vi "LookCANFileInfo.vi"(0 "Path输入":refnum<vi>, 1 "Language":u32, 2 "CAN报文统计":refnum<vi>, 3 "DBC数组":refnum<vi>) -> ()   [LabVIEW 2015]
panel:
  out "txtTile":string="CAN离线数据文件详细信息"
  out "文件信息":string
  out "报文统计":string[][](array[string])
  # "CAN离线数据文件详细信息"
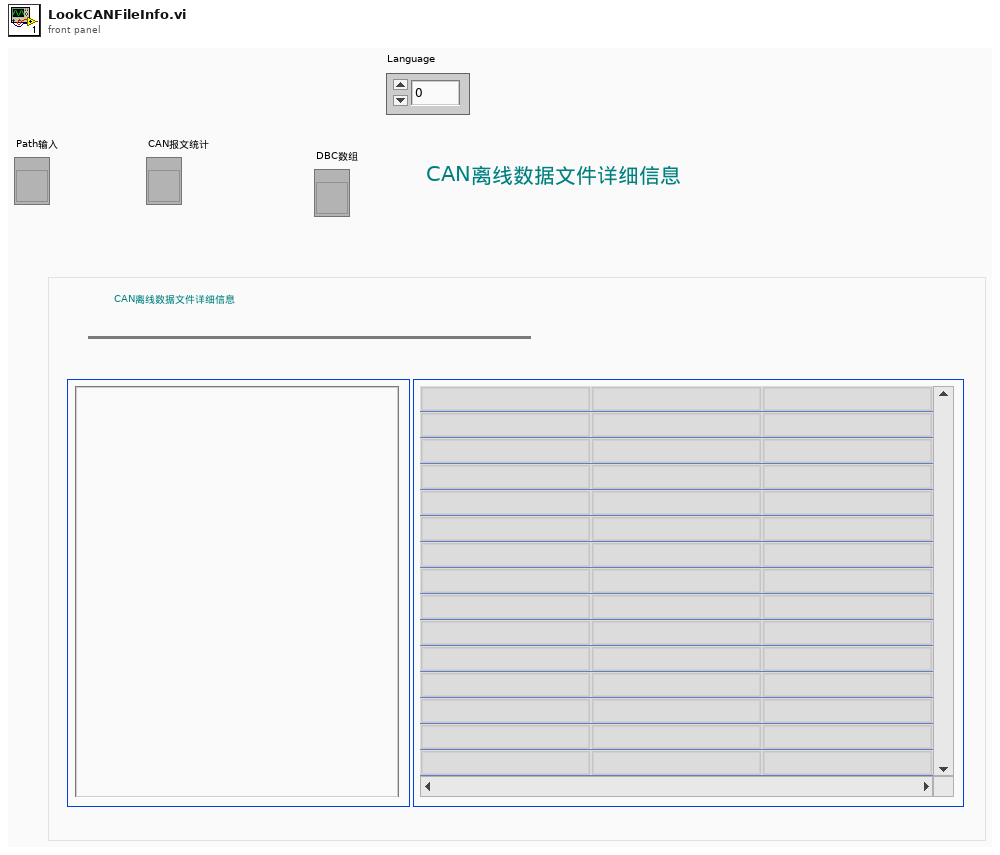
[diagram p1: front panel]
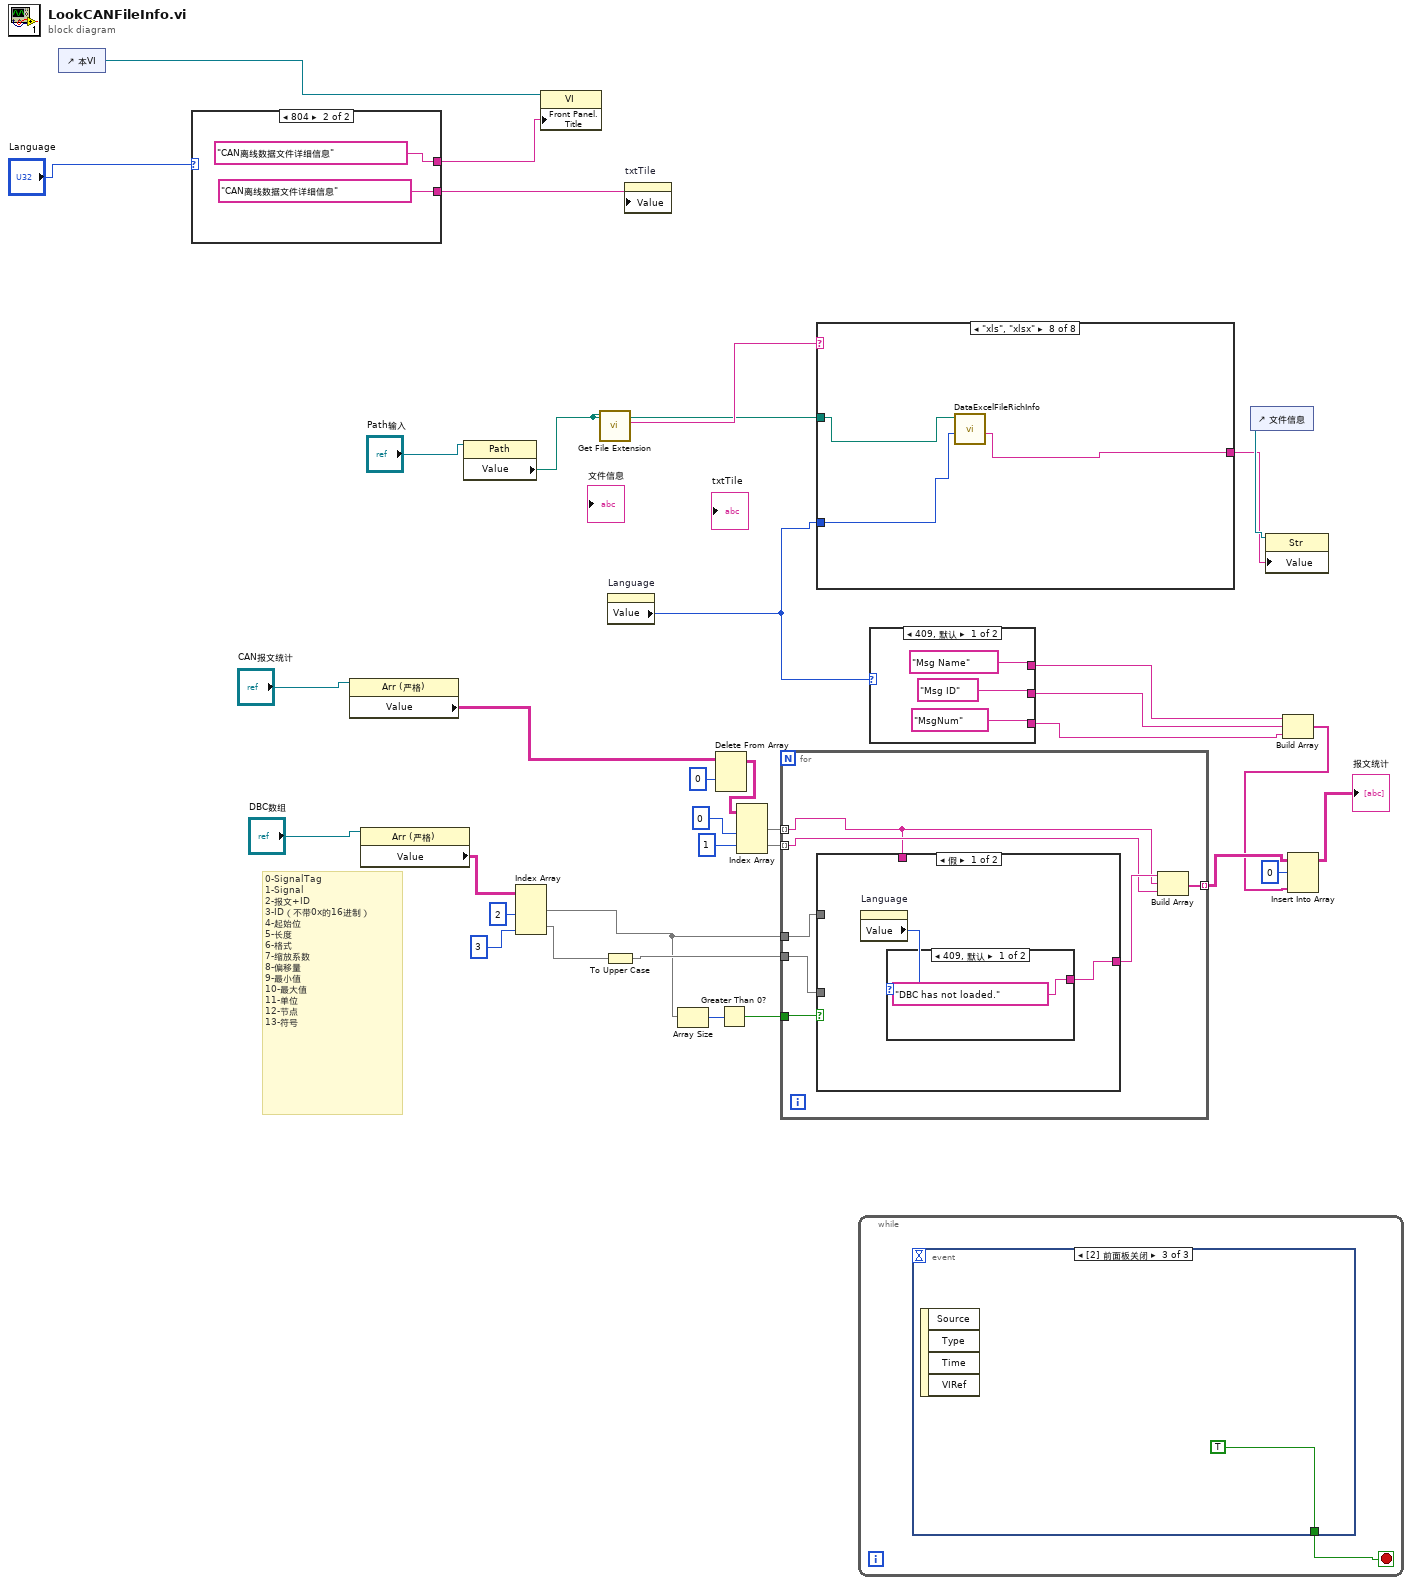
[diagram p0: block diagram]
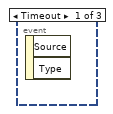
[diagram p2: hidden frame]
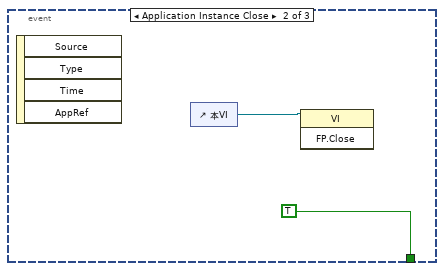
[diagram p3: hidden frame]
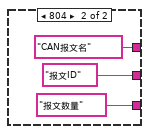
[diagram p4: hidden frame]
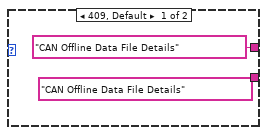
[diagram p5: hidden frame]
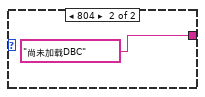
[diagram p6: hidden frame]
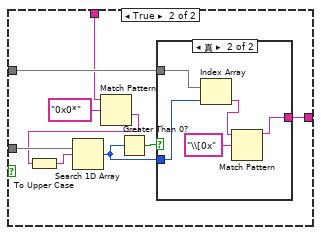
[diagram p7: hidden frame]
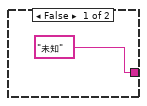
[diagram p8: hidden frame]
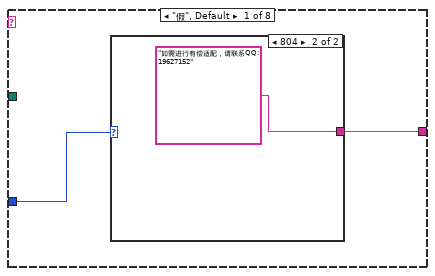
[diagram p9: hidden frame]
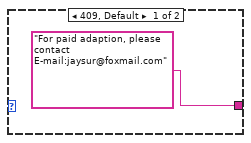
[diagram p10: hidden frame]
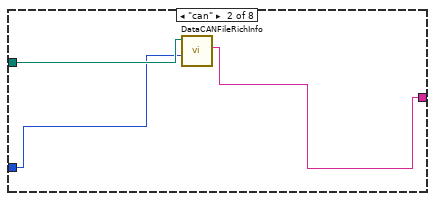
[diagram p11: hidden frame]
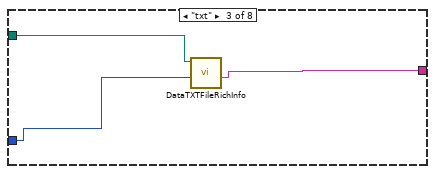
[diagram p12: hidden frame]
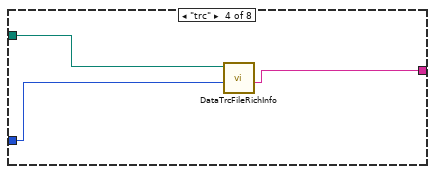
[diagram p13: hidden frame]
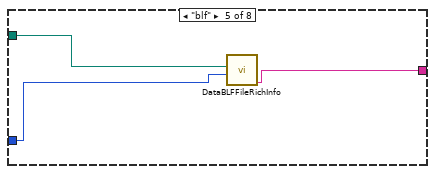
[diagram p14: hidden frame]
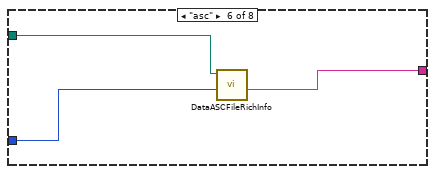
[diagram p15: hidden frame]
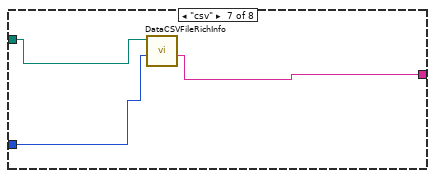
[diagram p16: hidden frame]
diagram:
  # "0-SignalTag\n1-Signal\n2-报文+ID\n3-ID（不带0x的16进制）\n4-起始位\n5-长度\n6-格式\n7-缩放系数\n8-偏移量\n9-最小值\n10-最大值\n11-单位\n12-节点\n13-符号"
  n1 = control-ref of="本VI"() -> (w2:refnum<vi>)
  n2 = case shown="804" "Language" {
    tunnel: ["CAN Offline Data File Details" "CAN离线数据文件详细信息"] -> w4
    tunnel: ["CAN Offline Data File Details" "CAN离线数据文件详细信息"] -> w1
    frame 409, Default {
    }
    frame 804 {
    }
  }
  n3 = property class="Arr (严格)"(reference="CAN报文统计") -> ("Value"=w23:string[][])  [unwired: 1 in, 2 out]
  n4 = property class="Arr (严格)"(reference="DBC数组") -> ("Value"=w27:string[][])  [unwired: 1 in, 2 out]
  n5 = property class="Path"(reference="Path输入") -> ("Value"=w31:path)  [unwired: 1 in, 2 out]
  n6 = Index Array(array=w27, index (col) #1=2 ("禁用的索引 (列)"), index (col) #2=3 ("索引 (列)")) -> (element #1=w20:string[], element #2=w22:string[])  [unwired: 2 in]
  n7 = property class="VI"(reference=w2, "Front Panel.Title"=w1) -> ()  [unwired: 1 in, 2 out]
  n8 = call <vilib>:"Get File Extension.vi"("file"=w31) -> ("lowercase file extension"=w32:string)  [unwired: 6 in, 4 out]
  n9 = To Upper Case(1:w22) -> (0:w21:string[])
  n10 = property on="Language" class="DigNum (严格)"() -> ("Value"=w3:u32)  [unwired: 2 in, 2 out]
  n11 = property on="txtTile" class="Str"("Value"=w4) -> ()  [unwired: 2 in, 2 out]
  n12 = Array Size(array=w20) -> (size(s)=w24:i32)
  n13 = Delete From Array(array=w23, index (row)=0 ("索引 (行)")) -> (array with subset deleted=w17:string[][])  [unwired: 2 in, 1 out]
  n14 = Greater Than 0?(x=w24) -> (x > 0?=w8:bool)
  n15 = Index Array(array=w17, index (col) #1=0 ("禁用的索引 (列)"), index (col) #2=1 ("索引 (列)")) -> (element #1=w14:string[], element #2=w13:string[])  [unwired: 2 in]
  n16 = for {
    tunnel: w14 -> [w39] mode=indexing
    tunnel: w13 -> [w41] mode=indexing
    tunnel: w20 -> [w45]
    tunnel: w21 -> [w44]
    tunnel: [w42] -> w12 mode=indexing
    tunnel: w8 -> [w40]
    n17 = case shown="假" w40 {
      tunnel: w45 -> [_ w58]
      tunnel: w44 -> [_ w57]
      tunnel: [w47 w56] -> w43
      tunnel: w39 -> [_ w54]
      frame False {
        n18 = property on="Language" class="DigNum (严格)"() -> ("Value"=w46:u32)  [unwired: 2 in, 2 out]
        n19 = case shown="409, 默认" w46 {
          tunnel: ["DBC has not loaded." "尚未加载DBC"] -> w47
          frame 409, Default {
          }
          frame 804 {
          }
        }
      }
      frame True {
        n20 = Match Pattern(string=w54, regular expression="0x0*" ("正则表达式")) -> (after substring=w50:string)  [unwired: 1 in, 3 out]
        n21 = To Upper Case(1:w50) -> (0:w51:string)
        n22 = Search 1D Array(1D array=w57, element=w51) -> (index of element=w52:i32)  [unwired: 1 in]
        n23 = Greater Than 0?(x=w52) -> (x > 0?=w55:bool)
        n24 = case shown="真" w55 {
          tunnel: w58 -> [_ w64]
          tunnel: ["未知" w61] -> w56
          tunnel: w52 -> [_ w63]
          frame False {
          }
          frame True {
            n25 = Index Array(array=w64, index=w63) -> (element=w62:string)
            n26 = Match Pattern(string=w62, regular expression="\\[0x" ("正则表达式")) -> (before substring=w61:string)  [unwired: 1 in, 3 out]
          }
        }
      }
    }
    n27 = Build Array(w43, w39, w41) -> (w42:string[])
  }
  n28 = case shown="\"xls\", \"xlsx\"" w32 {
    tunnel: w31 -> [_ w70 w74 w77 w79 w83 w86 w89]
    tunnel: [w66 w71 w73 w75 w78 w82 w85 w88] -> w29
    tunnel: w3 -> [w65 w69 w72 w76 w80 w81 w84 w87]
    frame "假", Default {
      n29 = case shown="804" w65 {
        tunnel: ["For paid adaption, please contact E-mail:jaysur@foxmail.com" "如需进行有偿适配，请联系QQ:19627152"] -> w66
        frame 409, Default {
        }
        frame 804 {
        }
      }
    }
    frame "can" {
      n30 = call "DataCANFileRichInfo.vi"("Language"=w69, "file path (dialog if empty)"=w70) -> ("FileInfo"=w71:string)  [unwired: 7 in, 2 out]
    }
    frame "txt" {
      n31 = call "DataTXTFileRichInfo.vi"("Language"=w72, "file path (dialog if empty)"=w74) -> ("FileInfo"=w73:string)  [unwired: 7 in, 2 out]
    }
    frame "trc" {
      n32 = call "DataTrcFileRichInfo.vi"("Language"=w76, "file path (dialog if empty)"=w77) -> ("FileInfo"=w75:string)  [unwired: 7 in, 2 out]
    }
    frame "blf" {
      n33 = call "DataBLFFileRichInfo.vi"("Language"=w80, "file path (dialog if empty)"=w79) -> ("FileInfo"=w78:string)  [unwired: 7 in, 2 out]
    }
    frame "asc" {
      n34 = call "DataASCFileRichInfo.vi"("Language"=w81, "file path (dialog if empty)"=w83) -> ("FileInfo"=w82:string)  [unwired: 7 in, 2 out]
    }
    frame "csv" {
      n35 = call "DataCSVFileRichInfo.vi"("Language"=w84, "file path (dialog if empty)"=w86) -> ("FileInfo"=w85:string)  [unwired: 7 in, 2 out]
    }
    frame "xls", "xlsx" {
      n36 = call "DataExcelFileRichInfo.vi"("Language"=w87, "file path (dialog if empty)"=w89) -> ("FileInfo"=w88:string)  [unwired: 7 in, 2 out]
    }
  }
  n37 = while {
    stop <- w90 stop-if-true
    n38 = event shown="[2] 前面板关闭" {
      selector: _ -> [_ _ _]
      dyn-events: _ -> [_ _ _]
      timeout: _ -> [_ _ _]
      tunnel: [_ TRUE TRUE] -> w90
      event Timeout {
        n39 = event-data() -> ()  [unwired: 1 in, 2 out]
      }
      event Application Instance Close {
        n40 = event-data() -> ()  [unwired: 1 in, 4 out]
        n41 = control-ref of="本VI"() -> (w92:refnum<vi>)
        n42 = invoke class="VI" method="FP.Close"(reference=w92) -> ()  [unwired: 2 in, 3 out]
      }
      event Panel Close {
        n43 = event-data() -> ()  [unwired: 1 in, 4 out]
      }
    }
  }
  n44 = case shown="409, 默认" w3 {
    tunnel: ["Msg Name" "CAN报文名"] -> w10
    tunnel: ["Msg ID" "报文ID"] -> w7
    tunnel: ["MsgNum" "报文数量"] -> w6
    frame 409, Default {
    }
    frame 804 {
    }
  }
  n45 = control-ref of="文件信息"() -> (w30:refnum<vi>)
  n46 = property class="Str"(reference=w30, "Value"=w29) -> ()  [unwired: 1 in, 2 out]
  n47 = Build Array(w10, w7, w6) -> (w9:string[])
  n48 = Insert Into Array(array=w12, index (row)=0 ("索引 (行)"), new element=w9) -> (→"报文统计":string[][])  [unwired: 1 in]
